vi "Stream from camera 1.vi"(1 "frame#":refnum<vi>, 2 "External Stop":refnum<vi>) -> ()   [LabVIEW 2013]
panel:
  out "overflow?":bool
  in  "ICImagingControl":refnum<k7>(container)
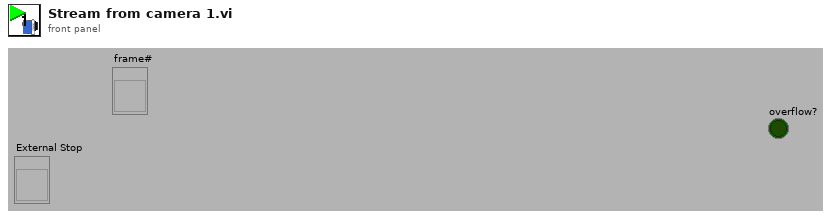
[diagram p1: front panel]
types:
  T1 = typedef "IMAQ Image.ctl" = refnum<image>
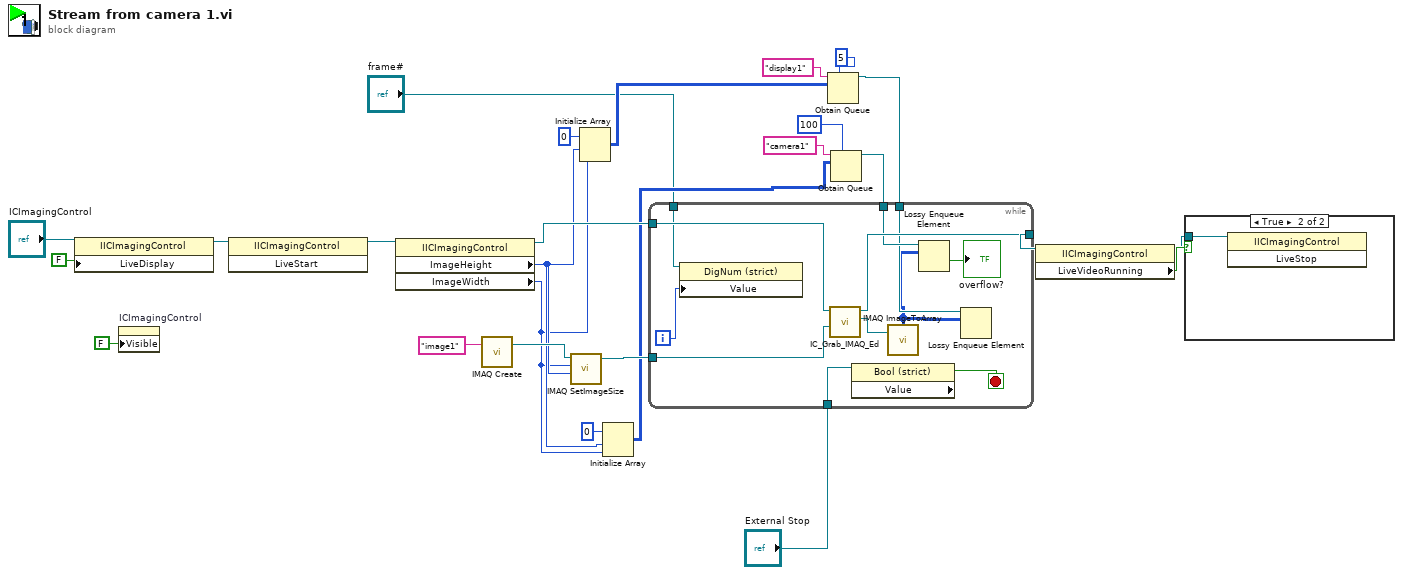
[diagram p0: block diagram]
diagram:
  n1 = property class="IICImagingControl"(reference="ICImagingControl", "LiveDisplay"=FALSE) -> (reference out=w24:refnum<k7>)  [unwired: 1 in, 1 out]
  n2 = property on="ICImagingControl" class="AXCont"("Visible"=FALSE) -> ()  [unwired: 2 in, 2 out]
  n3 = invoke class="IICImagingControl" method="LiveStart"(reference=w24) -> (reference out=w14:refnum<k7>)  [unwired: 2 in, 2 out]
  n4 = property class="IICImagingControl"(reference=w14) -> (reference out=w21:refnum<k7>, "ImageHeight"=w3:i32, "ImageWidth"=w2:i32)  [unwired: 1 in, 1 out]
  n5 = call "IMAQ Create"("Image Name"="image1") -> ("New Image"=w20:T1)  [unwired: 4 in, 1 out]
  n6 = call "IMAQ SetImageSize"("Y Resolution"=w3, "X Resolution"=w2, "Image"=w20) -> ("Image Out"=w18:T1)  [unwired: 2 in, 1 out]
  n7 = Initialize Array(u8 0 ("element"), w3, w2) -> (w4:u8[][])
  n8 = Initialize Array(i16 0 ("element"), w3, w2) -> (w9:i16[][])
  n9 = Obtain Queue(max queue size (-1, unlimited)=5, name (unnamed)="display1", element data type=w4) -> (queue out=w8:refnum<queue>)  [unwired: 2 in, 2 out]
  n10 = Obtain Queue(max queue size (-1, unlimited)=100, name (unnamed)="camera1", element data type=w9) -> (queue out=w17:refnum<queue>)  [unwired: 2 in, 2 out]
  n11 = while {
    tunnel: [w37] -> w23
    tunnel: w21 -> [w38]
    tunnel: w18 -> [w36]
    tunnel: w17 -> [w35]
    tunnel: "External Stop" -> [w32]
    tunnel: w8 -> [w31]
    tunnel: "frame#" -> [w27]
    i -> [w28]
    stop <- w33 stop-if-true
    n12 = property class="DigNum (strict)"(reference=w27, "Value"=w28) -> ()  [unwired: 1 in, 2 out]
    n13 = call "IC_Grab_IMAQ_Ed.vi"("Image Dest"=w36, "ICImagingControl In"=w38) -> ("Image Out"=w34:T1, "ICImagingControl Out"=w37:refnum<k7>)  [unwired: 2 in, 2 out]
    n14 = property class="Bool (strict)"(reference=w32) -> ("Value"=w33:bool)  [unwired: 1 in, 2 out]
    n15 = call "IMAQ ImageToArray"("Image"=w34) -> ("Image Pixels (U8)"=w29:u8[][])  [unwired: 3 in, 4 out]
    n16 = Lossy Enqueue Element(queue=w35, element=w29) -> (overflow?=→"overflow?":bool)  [unwired: 1 in, 3 out]
    n17 = Lossy Enqueue Element(queue=w31, element=w29) -> ()  [unwired: 1 in, 4 out]
  }
  n18 = property class="IICImagingControl"(reference=w23) -> (reference out=w22:refnum<k7>, "LiveVideoRunning"=w26:bool)  [unwired: 1 in, 1 out]
  n19 = case shown="True" w26 {
    tunnel: w22 -> [_ w39]
    frame False {
    }
    frame True {
      n20 = invoke class="IICImagingControl" method="LiveStop"(reference=w39) -> ()  [unwired: 2 in, 3 out]
    }
  }
